vi "Timer.vi"(0 "Timers_Start":bool[](array[boolean]), 2 "Wait_Time":dbl=10.0 format="%#_13g", 7 "Timer_Required":i32, 11 "Error_In":errorcluster, 13 "Timer_Select":T1=enum."Start_Timer") -> (4 "Timer_Time":dbl[](array[numeric]), 6 "Time_Out?":bool[](array[boolean]), 15 "Error_Out":errorcluster)   [LabVIEW 2023]
doc: "Used for time out opertion."
uses:
  Controls/Timer_Operation_Select.ctl
  Controls/Timer_Data.ctl
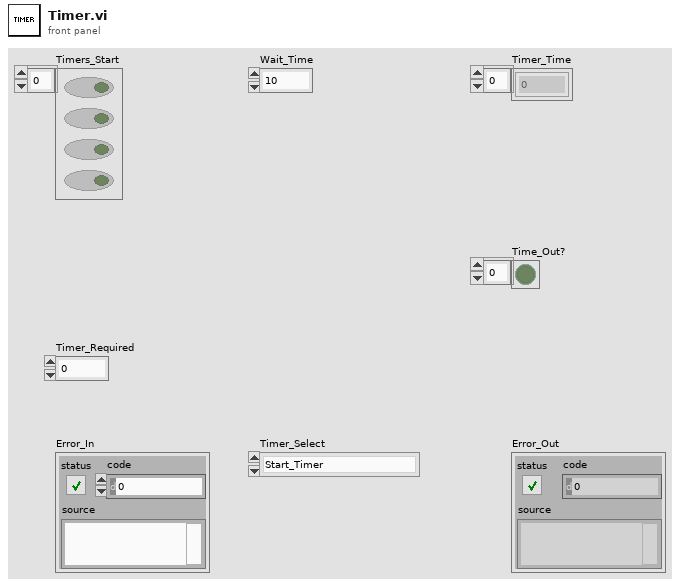
[diagram p1: front panel]
types:
  T1 = typedef "Timer_Operation_Select.ctl" = enum16{"Initialize", "Start_Timer", "Time_Out?", "Stop_Timer"}
  T2 = typedef "Timer_Data.ctl" = cluster{"T1_Start_Time":dbl[], "T_Start?":bool[], "Wait_Time":dbl}
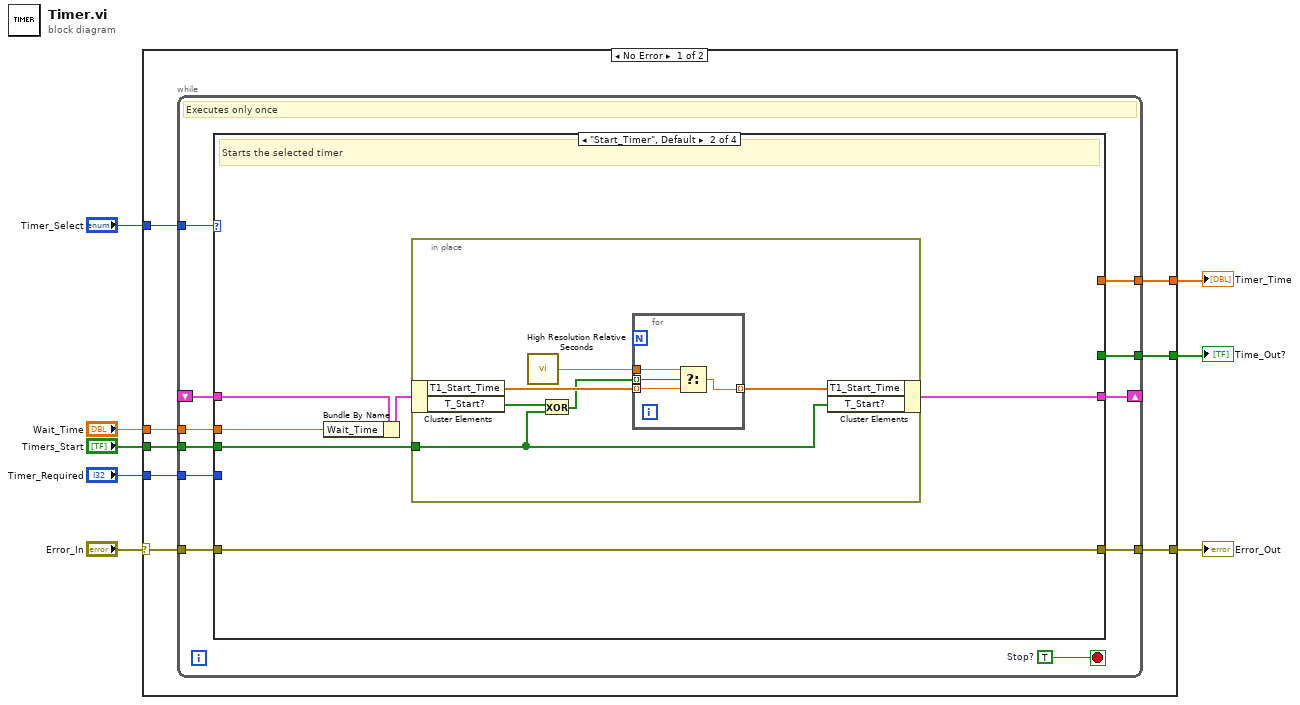
[diagram p0: block diagram]
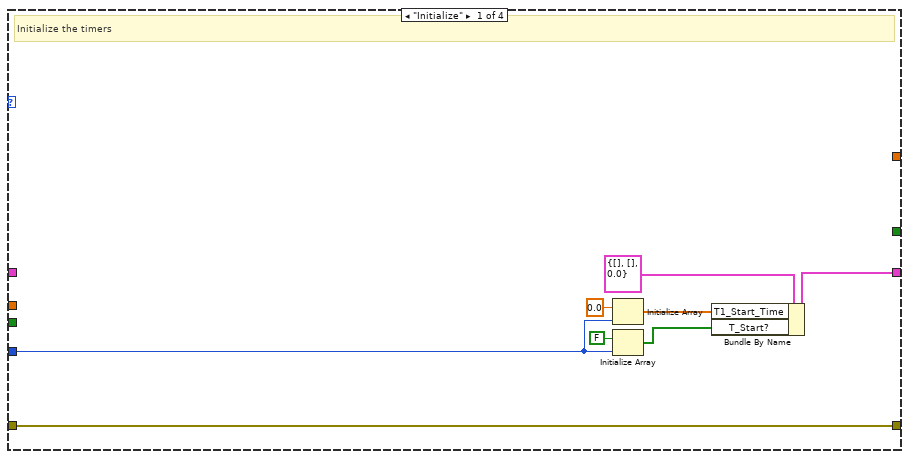
[diagram p2: hidden frame]
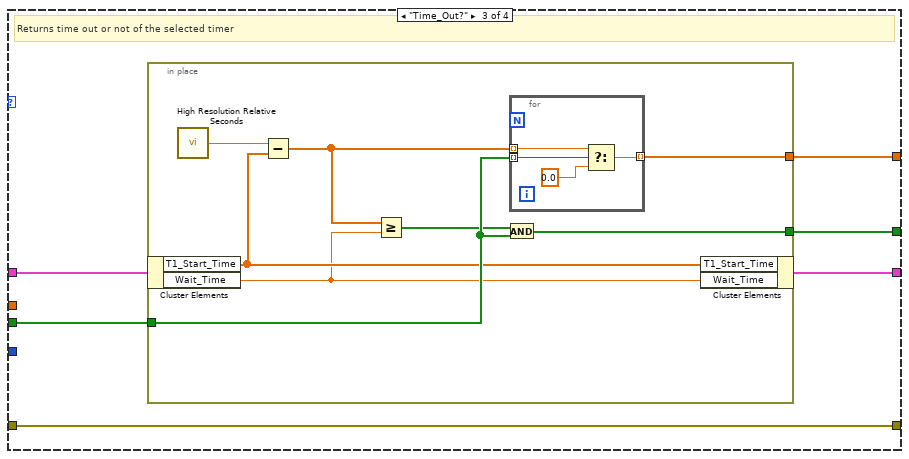
[diagram p3: hidden frame]
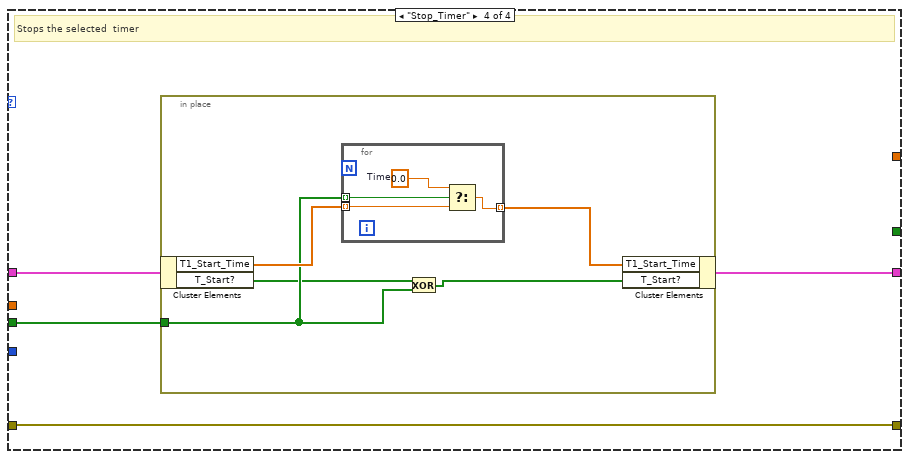
[diagram p4: hidden frame]
diagram:
  n1 = case shown="No Error" "Error_In" {
    selector: "Error_In" -> [w9 w83]
    tunnel: [w16 w83] -> w8
    tunnel: "Timer_Select" -> [w15 _]
    tunnel: "Wait_Time" -> [w14 _]
    tunnel: "Timers_Start" -> [w13 _]
    tunnel: [w12 _] -> w4
    tunnel: [w11 _] -> w3
    tunnel: "Timer_Required" -> [w10 _]
    frame No Error {
      n2 = while {
        tunnel: w9 -> [w26]
        tunnel: [w25] -> w16
        shift-right: [w22] -> _
        shift-left: _ -> [w24]
        tunnel: w15 -> [w23]
        tunnel: w14 -> [w21]
        tunnel: w13 -> [w20]
        tunnel: [w19] -> w12
        tunnel: [w18] -> w11
        tunnel: w10 -> [w17]
        stop <- w27 stop-if-true
        w27 = TRUE  # Stop?
        # "Executes only once"
        n3 = case shown="\"Start_Timer\", Default" w23 {
          tunnel: w26 -> [w35 w36 w52 w70]
          tunnel: [w35 w36 w52 w70] -> w25
          tunnel: w24 -> [_ w39 w56 w72]
          tunnel: [w34 w41 w57 w73] -> w22
          tunnel: w21 -> [_ w40 _ _]
          tunnel: w20 -> [_ w37 w55 w71]
          tunnel: [_ _ w54 _] -> w19
          tunnel: [_ _ w53 _] -> w18
          tunnel: w17 -> [w29 _ _ _]
          frame "Initialize" {
            # "Initialize the timers"
            n4 = Initialize Array(0.0 ("element"), w29) -> (w32:dbl[])
            n5 = Initialize Array(FALSE, w29) -> (w30:bool[])
            n6 = Bundle By Name(cluster=T2 {"T1_Start_Time"=[], "T_Start?"=[], "Wait_Time"=0.0} ("Timer_Data"), "T1_Start_Time"=w32, "T_Start?"=w30) -> (w34:T2)
          }
          frame "Start_Timer", Default {
            # "Starts the selected timer"
            n7 = Bundle By Name(cluster=w39, "Wait_Time"=w40) -> (w38:T2)
            n8 = in-place {
              in-place-border: w37 -> [w42]
              n9 = in-place-cluster #1(w38) -> ("T1_Start_Time"=w47:dbl[], "T_Start?"=w44:bool[])
              n10 = call <vilib>:"High Resolution Relative Seconds.vi"() -> ("relative seconds"=w45:dbl)
              n11 = Exclusive Or(1:w42, 2:w44) -> (0:w43:bool[])
              n12 = for {
                tunnel: w47 -> [w51] mode=indexing
                tunnel: [w50] -> w46 mode=indexing
                tunnel: w45 -> [w49]
                tunnel: w43 -> [w48] mode=indexing
                n13 = Select(t=w49, s=w48, f=w51) -> (s? t:f=w50:dbl)
              }
              n14 = in-place-cluster #1("T1_Start_Time"=w46, "T_Start?"=w42) -> (w41:T2)
            }
          }
          frame "Time_Out?" {
            # "Returns time out or not of the selected timer"
            n15 = in-place {
              in-place-border: [w65] -> w54
              in-place-border: [w64] -> w53
              in-place-border: w55 -> [w63]
              n16 = in-place-cluster #2(w56) -> ("T1_Start_Time"=w62:dbl[], "Wait_Time"=w61:dbl)
              n17 = call <vilib>:"High Resolution Relative Seconds.vi"() -> ("relative seconds"=w60:dbl)
              n18 = Subtract(x=w60, y=w62) -> (x-y=w59:dbl[])
              n19 = Greater Or Equal?(x=w59, y=w61) -> (x >= y?=w58:bool[])
              n20 = And(x=w58, y=w63) -> (x .and. y?=w65:bool[])
              n21 = for {
                tunnel: [w69] -> w64 mode=indexing
                tunnel: w63 -> [w68] mode=indexing
                tunnel: w59 -> [w67] mode=indexing
                n22 = Select(t=w67, s=w68, f=0.0) -> (s? t:f=w69:dbl)
              }
              n23 = in-place-cluster #2("T1_Start_Time"=w62, "Wait_Time"=w61) -> (w57:T2)
            }
          }
          frame "Stop_Timer" {
            # "Stops the selected  timer"
            n24 = in-place {
              in-place-border: w71 -> [w75]
              n25 = in-place-cluster #3(w72) -> ("T1_Start_Time"=w78:dbl[], "T_Start?"=w74:bool[])
              n26 = for {
                tunnel: w78 -> [w81] mode=indexing
                tunnel: [w80] -> w77 mode=indexing
                tunnel: w75 -> [w79] mode=indexing
                w82 = 0.0  # Time
                n27 = Select(t=w82, s=w79, f=w81) -> (s? t:f=w80:dbl)
              }
              n28 = Exclusive Or(1:w75, 2:w74) -> (0:w76:bool[])
              n29 = in-place-cluster #3("T1_Start_Time"=w77, "T_Start?"=w76) -> (w73:T2)
            }
          }
        }
      }
    }
    frame Error {
    }
  }
  "Error_Out" <- w8
  "Timer_Time" <- w3
  "Time_Out?" <- w4
